vi "IQ to XY Cluster.vi"(1 "wfm data":waveform(cdb)) -> (0 "xy cluster":cluster{"Array":dbl[], "Array":dbl[]})   [LabVIEW 2021]
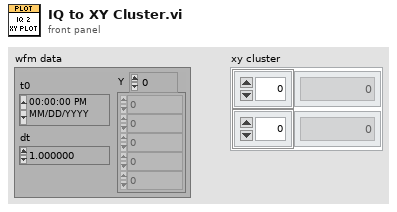
[diagram p1: front panel]
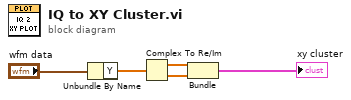
[diagram p0: block diagram]
diagram:
  n1 = Unbundle By Name("wfm data") -> ("Y"=w2:cdb[])
  n2 = Complex To Re/Im(x + iy=w2) -> (x=w3:dbl[], y=w4:dbl[])
  n3 = Bundle(w3, w4) -> (→"xy cluster":cluster{dbl[], dbl[]})  [unwired: 1 in]
